vi "ReadConfigFile.vi"(0 "path to config file":path) -> (1 "zstop to calibration origin":dbl[](array[numeric]) format="%#_10g", 2 "rel. location of calibration points":dbl[][](array[numeric]), 3 "zstop to first module corners":dbl[][](array[numeric]) format="%#_10g", 4 "error out":errorcluster)   [LabVIEW 2016]
doc: "Reads a stave configuration file."
panel:
  in  "Array":dbl[][](array[numeric])
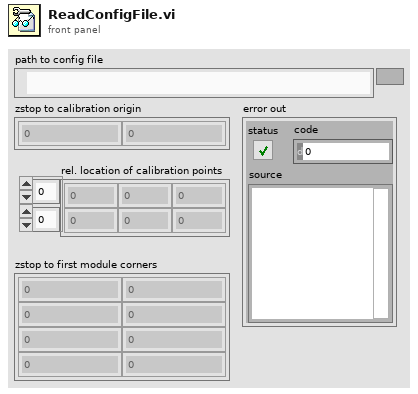
[diagram p1: front panel]
types:
  T1 = cluster{"[0]":cluster{dbl[]}, "[1]":cluster{dbl[]}, "[2]":cluster{dbl[]}, "[3]":cluster{dbl[]}, "[4]":cluster{dbl[]}, "[5]":cluster{dbl[]}}
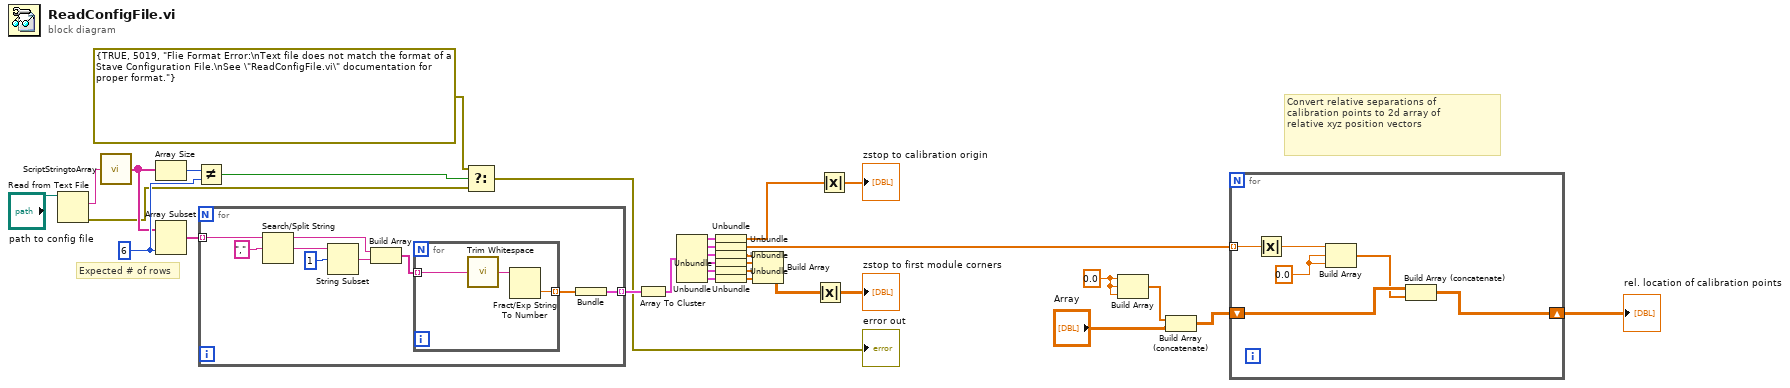
[diagram p0: block diagram]
diagram:
  w4 = 0.0 ("element")
  w27 = 6
  # "Convert relative separations of\ncalibration points to 2d array of\nrelative xyz position vectors"
  # "Expected # of rows"
  n1 = Read from Text File(file (use dialog)="path to config file") -> (text=w31:string, error out=w10:errorcluster)  [unwired: 3 in, 2 out]
  n2 = call "ScriptStringtoArray.vi"("spreadsheet string"=w31) -> ("Array"=w26:string[])
  n3 = Array Size(array=w26) -> (size(s)=w30:i32)
  n4 = Array Subset(array=w26, length=w27) -> (w25:string[])  [unwired: 1 in]
  n5 = Not Equal?(x=w30, y=w27) -> (x != y?=w29:bool)
  n6 = for {
    tunnel: w25 -> [w41] mode=indexing
    tunnel: [w33] -> w24 mode=indexing
    n7 = Search/Split String(string=w41, search string/char (-)=",") -> (substring before match=w36:string, match + rest of string=w38:string)  [unwired: 1 in, 1 out]
    n8 = String Subset(string=w38, offset (0)=1) -> (substring=w37:string)  [unwired: 1 in]
    n9 = Build Array(w36, w37) -> (w35:string[])
    n10 = for {
      tunnel: w35 -> [w44] mode=indexing
      tunnel: [w42] -> w34 mode=indexing
      n11 = call <vilib>:"Trim Whitespace.vi"("string"=w44) -> ("trimmed string"=w43:string)  [unwired: 1 in]
      n12 = Fract/Exp String To Number(string=w43) -> (number=w42:dbl)  [unwired: 3 in, 1 out]
    }
    n13 = Bundle(w34) -> (w33:cluster{dbl[]})  [unwired: 1 in]
  }
  n14 = Select(t=errorcluster {TRUE, 5019, "Flie Format Error:\nText file does not match the format of a Stave Configuration File.\nSee \"ReadConfigFile.vi\" documentation for proper format."}, s=w29, f=w10) -> (s? t:f=→"error out":errorcluster)
  n15 = Array To Cluster(array=w24) -> (cluster=w23:T1)
  n16 = Unbundle(w23) -> ("[0]"=w22:cluster{dbl[]}, "[1]"=w21:cluster{dbl[]}, "[2]"=w20:cluster{dbl[]}, "[3]"=w19:cluster{dbl[]}, "[4]"=w18:cluster{dbl[]}, "[5]"=w17:cluster{dbl[]})
  n17 = Unbundle(w22) -> (w7:dbl[])
  n18 = Unbundle(w21) -> (w9:dbl[])
  n19 = Unbundle(w20) -> (w11:dbl[])
  n20 = Unbundle(w19) -> (w16:dbl[])
  n21 = Unbundle(w18) -> (w15:dbl[])
  n22 = Unbundle(w17) -> (w14:dbl[])
  n23 = Build Array(w11, w16, w15, w14) -> (w13:dbl[][])
  n24 = Absolute Value(x=w13) -> (abs(x)=→"zstop to first module corners":dbl[][])
  n25 = Absolute Value(x=w7) -> (abs(x)=→"zstop to calibration origin":dbl[])
  n26 = Build Array(w4, w4, w4) -> (w2:dbl[])
  n27 = Build Array (concatenate)(w2, "Array") -> (w1:dbl[][])
  n28 = for {
    tunnel: w9 -> [w46] mode=indexing
    shift-right: [w47] -> w8
    shift-left: w1 -> [w49]
    w50 = 0.0 ("element")
    n29 = Absolute Value(x=w46) -> (abs(x)=w45:dbl)
    n30 = Build Array(w45, w50, w50) -> (w48:dbl[])
    n31 = Build Array (concatenate)(w49, w48) -> (w47:dbl[][])
  }
  "rel. location of calibration points" <- w8
